vi "Untitled 3.vi"() -> ()   [LabVIEW 2015]
panel:
  in  "stop 2":bool
  in  "stop":bool
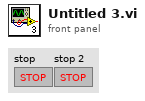
[diagram p1: front panel]
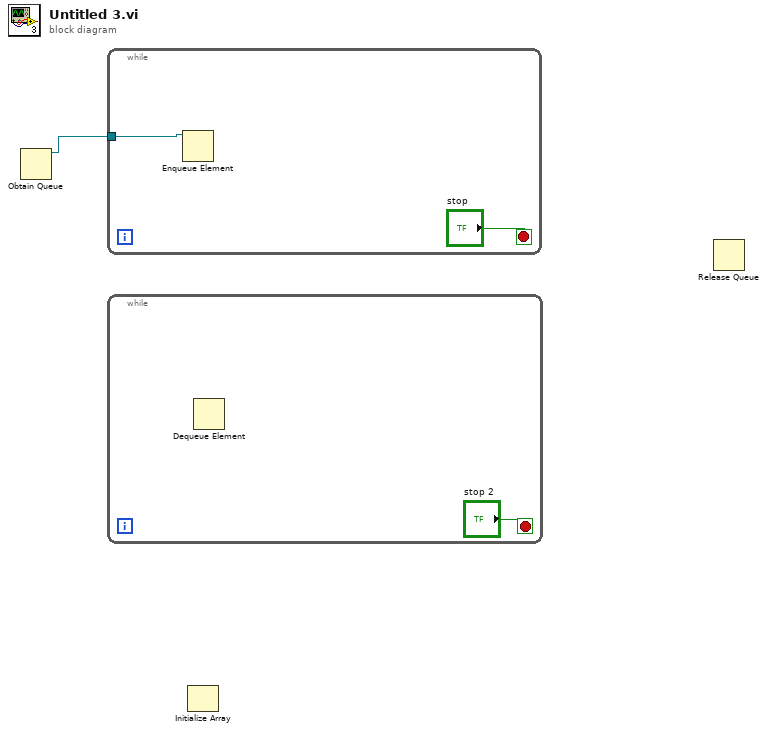
[diagram p0: block diagram]
diagram:
  n1 = Obtain Queue() -> (queue out=w1:refnum<queue>)  [unwired: 5 in, 2 out]
  n2 = while {
    tunnel: w1 -> [w3]
    stop <- "stop" stop-if-true
    n3 = Enqueue Element(queue=w3) -> ()  [unwired: 3 in, 3 out]
  }
  n4 = while {
    stop <- "stop 2" stop-if-true
    n5 = Dequeue Element() -> ()  [unwired: 3 in, 4 out]
  }
  n6 = Initialize Array() -> ()  [unwired: 2 in, 1 out]
  n7 = Release Queue() -> ()  [unwired: 3 in, 3 out]
